vi "Update Exp Time Abs Control.vi"(8 "error in (no error)":errorcluster, 11 "Camera Quick Settings Panel in":refnum<class "Camera Quick Settings Panel.lvclass">) -> (0 "error out":errorcluster, 3 "Camera Quick Settings Panel out":refnum<class "Camera Quick Settings Panel.lvclass">)   [LabVIEW 2014, in "Camera Quick Settings Panel.lvlib" / "Camera Quick Settings Panel.lvclass"]
uses:
  Camera Quick Settings Panel.lvclass
  Camera Quick Settings Panel.lvclass/Camera Quick Settings Panel.ctl
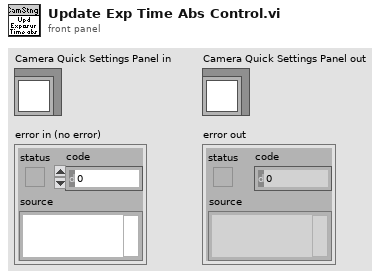
[diagram p1: front panel]
types:
  T1 = cluster{"U32 Value Control":refnum<vi>, "DBL Value Control":refnum<vi>, "String Value Control":refnum<vi>, "Enum Value Control":refnum<vi>, "Boolean Value Control":refnum<vi>, "Command Value Control":refnum<vi>}
  T2 = typedef "IMAQdx.ctl" = refnum<k21>
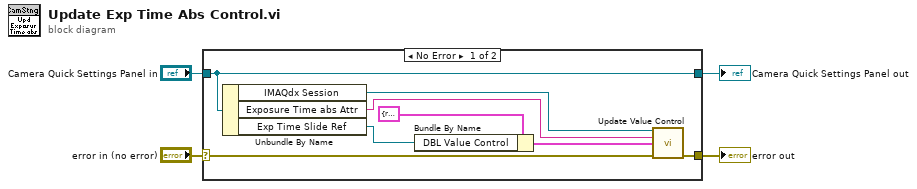
[diagram p0: block diagram]
diagram:
  n1 = case shown="No Error" "error in (no error)" {
    selector: "error in (no error)" -> [w9 w14]
    tunnel: [w8 w14] -> w3
    tunnel: [w12 w13] -> w1
    tunnel: "Camera Quick Settings Panel in" -> [w12 w13]
    frame No Error {
      n2 = Unbundle By Name(w12) -> ("IMAQdx Session"=w10:T2, "Exposure Time abs Attr"=w11:string, "Exp Time Slide Ref"=w5:refnum<vi>)
      n3 = Bundle By Name(cluster=T1 {"U32 Value Control"=refnum, "DBL Value Control"=refnum, "String Value Control"=refnum, "Enum Value Control"=refnum, "Boolean Value Control"=refnum, "Command Value Control"=refnum} ("Tab Control Ref In"), "DBL Value Control"=w5) -> (w6:T1)
      n4 = call "Update Value Control.vi"("Session In"=w10, "Active Item:Tag"=w11, "Tab Control Ref In"=w6, "error in (no error)"=w9) -> ("error out"=w8:errorcluster)  [unwired: 10 in, 1 out]
    }
    frame Error {
    }
  }
  "error out" <- w3
  "Camera Quick Settings Panel out" <- w1
